vi "Read Stop When Parent Stopped.vi"(11 "Base Actor in":refnum<class "Base Actor.lvclass">) -> (2 "Stop When Parent Stopped":bool)   [LabVIEW 2025, in "jettl.lvlib" / "Actor.lvlib" / "Base Actor.lvclass"]
uses:
  Base Actor.lvclass
  Base Actor.lvclass/Base Actor.ctl
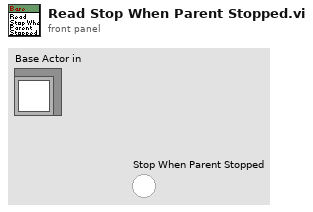
[diagram p1: front panel]
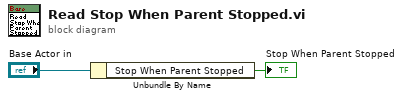
[diagram p0: block diagram]
diagram:
  n1 = Unbundle By Name("Base Actor in") -> ("Stop When Parent Stopped"=→"Stop When Parent Stopped":bool)
